vi "Load node UI optimized.vi"(8 "error in":errorcluster, 10 "node":T11, 11 "state in":T1) -> (0 "error out":errorcluster, 3 "state out":T1)   [LabVIEW 2014, in "Standard Editor.lvlib"]
doc: "This VI will insert the UI from a node into a subpanel."
uses:
  Standard Editor.lvlib
  <vilib>/NI/Configuration Framework/Node/NodeRef.ctl
  <vilib>/NI/Configuration Framework/Node/NISE_CEF_Node.lvclass
  Controls/StateCluster.ctl
  Configuration Editor/Classes/SystemConfigRepo/SystemConfigRepo.lvclass
  Configuration Editor/Classes/Systems/Systems.lvclass
  <vilib>/NI/Configuration Framework/Node/StandardEvents.ctl
  <vilib>/NI/Configuration Framework/Node/UserEventRef.ctl
  <vilib>/NI/Configuration Framework/Controls/EventCluster.ctl
  <vilib>/NI/Configuration Framework/Node/NodeChangeEvent.ctl
  <vilib>/NI/Configuration Framework/Node/CacheState.ctl
  <vilib>/NI/Configuration Framework/Node/RefreshUIEvent.ctl
  <vilib>/NI/Configuration Framework/Node/StopEvent.ctl
  <vilib>/NI/Configuration Framework/glyph manager/glyph manager.ctl
  <vilib>/picture/picture.llb/imagedata.ctl
  <vilib>/NI/AMC/Message Queue.ctl
  <vilib>/NI/AMC/Message.ctl
  <vilib>/NI/Tools/Keyed Array/KeyedArray.ctl
  <vilib>/NI/Tools/Keyed Array/Tools_KeyedArray.lvlib
  <vilib>/NI/AMC/AMC.lvlib
  <vilib>/NI/Configuration Framework/NISE_CEF_TreeControl.lvlib
  <vilib>/NI/Configuration Framework/glyph manager/glyph manager.lvlib
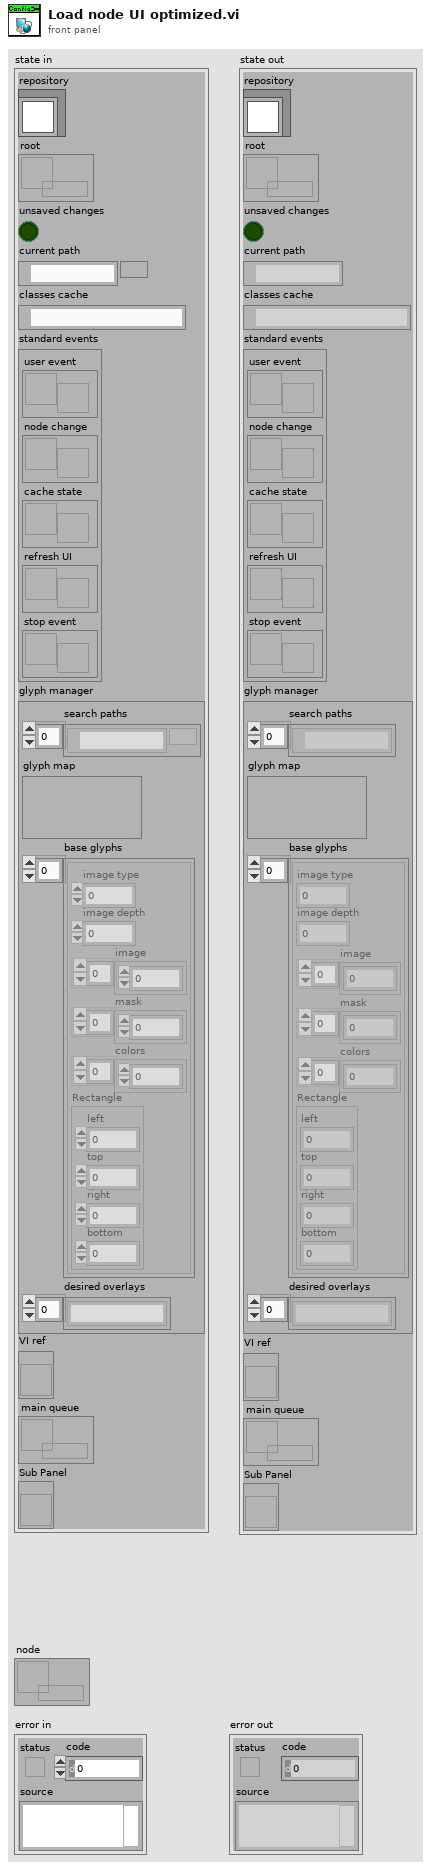
[diagram p1: front panel]
types:
  T1 = typedef "Standard Editor.lvlib/StateCluster.ctl" = cluster{"repository":refnum<class "SystemConfigRepo.lvclass">, "root":refnum<data-value>, "unsaved changes":bool, "current path":path, "classes cache":path, "standard events":T2, "glyph manager":T8, "VI ref":refnum<vi>, "main queue":T10, "Sub Panel":refnum<vi>}
  T2 = typedef "NISE_CEF_Node.lvclass/StandardEvents.ctl" = cluster{"user event":T3, "node change":T4, "cache state":T5, "refresh UI":T6, "stop event":T7}
  T3 = typedef "NISE_CEF_Node.lvclass/UserEventRef.ctl" = refnum<user-event>
  T4 = typedef "NISE_CEF_Node.lvclass/NodeChangeEvent.ctl" = refnum<user-event>
  T5 = typedef "NISE_CEF_Node.lvclass/CacheState.ctl" = refnum<user-event>
  T6 = typedef "NISE_CEF_Node.lvclass/RefreshUIEvent.ctl" = refnum<user-event>
  T7 = typedef "NISE_CEF_Node.lvclass/StopEvent.ctl" = refnum<user-event>
  T8 = typedef "glyph manager.lvlib/glyph manager.ctl" = cluster{"search paths":path[], "glyph map":variant, "base glyphs":T9[], "desired overlays":string[]}
  T9 = typedef "imagedata.ctl" = cluster{"image type":i32, "image depth":i32, "image":u8[], "mask":u8[], "colors":u32[], "Rectangle":cluster{"left":i16, "top":i16, "right":i16, "bottom":i16}}
  T10 = typedef "AMC.lvlib/Message Queue.ctl" = refnum<queue>
  T11 = typedef "NISE_CEF_Node.lvclass/NodeRef.ctl" = refnum<data-value>
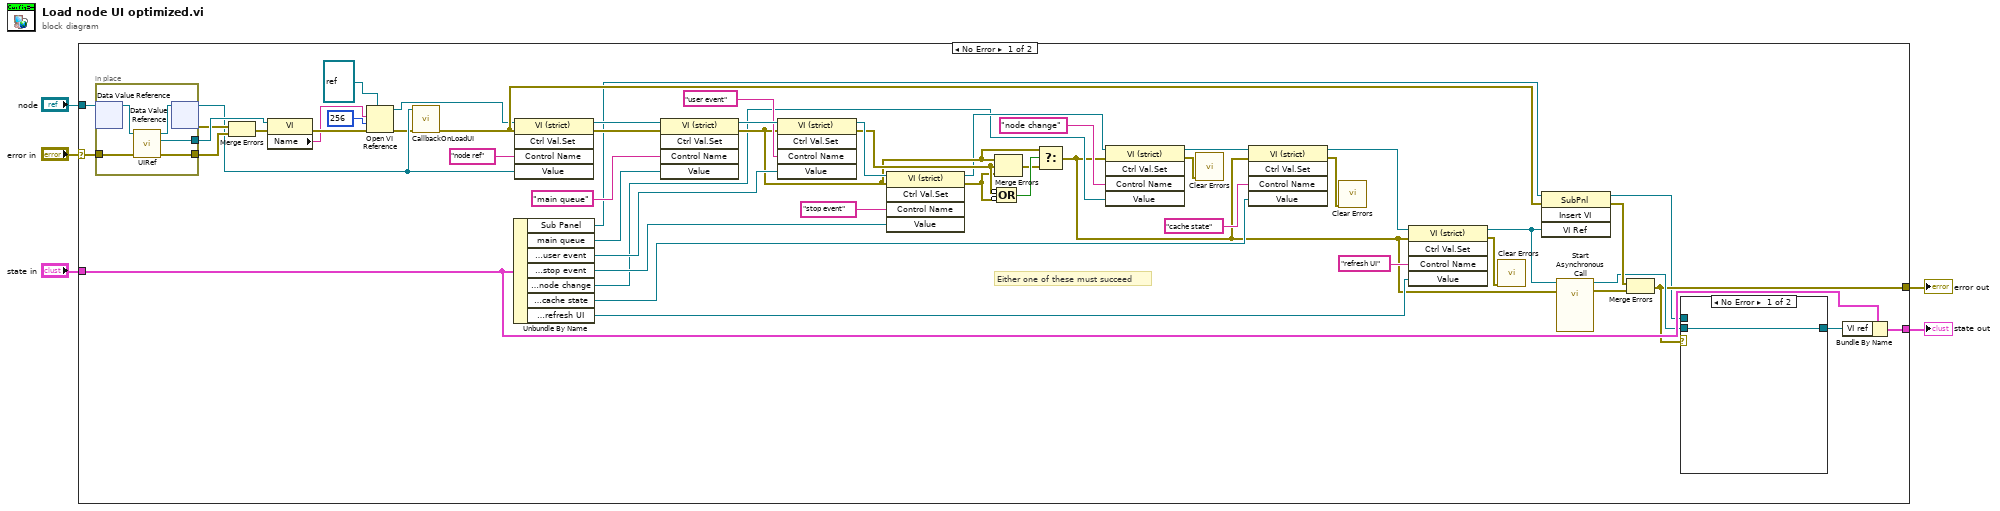
[diagram p0: block diagram]
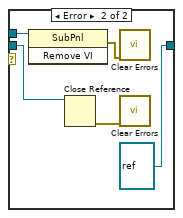
[diagram p2: hidden frame]
diagram:
  n1 = case shown="No Error" "error in" {
    selector: "error in" -> [w52 w71]
    tunnel: [w7 w71] -> w4
    tunnel: "node" -> [w50 _]
    tunnel: "state in" -> [w13 w70]
    tunnel: [w12 w70] -> w1
    frame No Error {
      # "Either one of these must succeed"
      n2 = in-place {
        in-place-border: w52 -> [w66]
        in-place-border: [w67] -> w51
        in-place-border: [w65] -> w49
        n3 = in-place-dvr #1(w50) -> (w69:refnum<class "NISE_CEF_Node.lvclass">)  [unwired: 1 out]
        n4 = call-dynamic "UIRef.vi"("error in"=w66, "node in"=w69) -> ("error out"=w65:errorcluster, "VI refnum"=w67:refnum<vi>, "node out"=w68:refnum<class "NISE_CEF_Node.lvclass">)  [unwired: 7 in]
        n5 = in-place-dvr #1(w68) -> (w24:T11, w48:errorcluster)
      }
      n6 = Merge Errors(w48, w49) -> (w47:errorcluster)
      n7 = property class="VI"(reference=w51, error in=w47) -> (error out=w25:errorcluster, "Name"=w18:string)  [unwired: 1 out]
      n8 = Open VI Reference(type specifier VI Refnum (for type only)=refnum<vi> refnum, vi path=w18, options=256, error in (no error)=w25) -> (vi reference=w15:refnum<vi>, error out=w19:errorcluster)  [unwired: 2 in]
      n9 = call <vilib>:"CallbackOnLoadUI.vi"("error in"=w19, "node"=w24) -> ("error out"=w22:errorcluster)  [unwired: 9 in]
      n10 = Unbundle By Name(w13) -> ("Sub Panel"=w11:refnum<vi>, "main queue"=w14:T10, "standard events.user event"=w46:T3, "standard events.stop event"=w44:T7, "standard events.node change"=w31:T4, "standard events.cache state"=w30:T5, "standard events.refresh UI"=w29:T6)
      n11 = invoke class="VI (strict)" method="Ctrl Val.Set"(reference=w15, error in=w22, "Control Name"="node ref", "Value"=w24) -> (reference out=w56:refnum<vi>, error out=w55:errorcluster)  [unwired: 1 in, 3 out]
      n12 = invoke class="VI (strict)" method="Ctrl Val.Set"(reference=w56, error in=w55, "Control Name"="main queue", "Value"=w14) -> (reference out=w54:refnum<vi>, error out=w38:errorcluster)  [unwired: 1 in, 3 out]
      n13 = invoke class="VI (strict)" method="Ctrl Val.Set"(reference=w54, error in=w38, "Control Name"="user event", "Value"=w46) -> (reference out=w45:refnum<vi>, error out=w42:errorcluster)  [unwired: 1 in, 3 out]
      n14 = invoke class="VI (strict)" method="Ctrl Val.Set"(reference=w45, error in=w38, "Control Name"="stop event", "Value"=w44) -> (reference out=w37:refnum<vi>, error out=w41:errorcluster)  [unwired: 1 in, 3 out]
      n15 = Merge Errors(w38, w42, w41) -> (w39:errorcluster)
      n16 = Compound Arithmetic op=OR(invert w42, invert w41) -> (w40:bool)
      n17 = Select(t=w38, s=w40, f=w39) -> (s? t:f=w21:errorcluster)
      n18 = invoke class="VI (strict)" method="Ctrl Val.Set"(reference=w37, error in=w21, "Control Name"="node change", "Value"=w31) -> (reference out=w36:refnum<vi>, error out=w27:errorcluster)  [unwired: 1 in, 3 out]
      n19 = call <vilib>:"Clear Errors.vi"("error in (no error)"=w27) -> ()  [unwired: 5 in, 2 out]
      n20 = invoke class="VI (strict)" method="Ctrl Val.Set"(reference=w36, error in=w21, "Control Name"="cache state", "Value"=w30) -> (reference out=w35:refnum<vi>, error out=w28:errorcluster)  [unwired: 1 in, 3 out]
      n21 = call <vilib>:"Clear Errors.vi"("error in (no error)"=w28) -> ()  [unwired: 5 in, 2 out]
      n22 = invoke class="VI (strict)" method="Ctrl Val.Set"(reference=w35, error in=w21, "Control Name"="refresh UI", "Value"=w29) -> (reference out=w23:refnum<vi>, error out=w26:errorcluster)  [unwired: 1 in, 3 out]
      n23 = call <vilib>:"Clear Errors.vi"("error in (no error)"=w26) -> ()  [unwired: 5 in, 2 out]
      n24 = invoke class="SubPnl" method="Insert VI"(reference=w11, error in=w22, "VI Ref"=w23) -> (reference out=w6:refnum<vi>, error out=w20:errorcluster)  [unwired: 1 in, 2 out]
      n25 = call-by-ref "Start Asynchronous Call"(reference=w23, error in=w21) -> (reference out=w9:refnum<vi>, error out=w10:errorcluster)  [unwired: 12 in]
      n26 = Merge Errors(w20, w10) -> (w7:errorcluster)
      n27 = case shown="No Error" w7 {
        tunnel: w9 -> [w59 w62]
        tunnel: [w59 refnum<vi> refnum ("type specifier VI Refnum (for type only)")] -> w8
        tunnel: w6 -> [_ w60]
        frame No Error {
        }
        frame Error {
          n28 = invoke class="SubPnl" method="Remove VI"(reference=w60) -> (error out=w61:errorcluster)  [unwired: 2 in, 2 out]
          n29 = Close Reference(reference=w62) -> (error out=w64:errorcluster)  [unwired: 1 in]
          n30 = call <vilib>:"Clear Errors.vi"("error in (no error)"=w61) -> ()  [unwired: 5 in, 2 out]
          n31 = call <vilib>:"Clear Errors.vi"("error in (no error)"=w64) -> ()  [unwired: 5 in, 2 out]
        }
      }
      n32 = Bundle By Name(cluster=w13, "VI ref"=w8) -> (w12:T1)
    }
    frame Error {
    }
  }
  "error out" <- w4
  "state out" <- w1
